vi "Translator.GatherControls.Prepare.vi"(8 "error in":errorcluster, 9 "root":string, 10 "Controls in":refnum<vi>[](array[refnum])) -> (0 "error out":errorcluster, 2 "Controls out":T1[](array[typedef]))   [LabVIEW 2016]
uses:
  Translator.ControlData.ctl
  Translator.ControlTypes.ctl
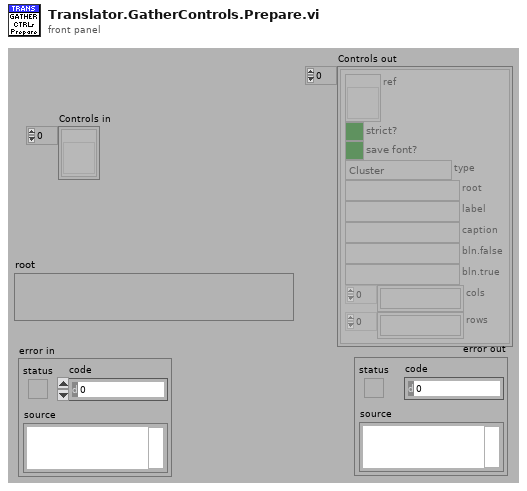
[diagram p1: front panel]
types:
  T1 = typedef "Translator.ControlData.ctl" = cluster{"ref":refnum<vi>, "strict?":bool, "save font?":bool, "type":T2, "root":string, "label":string, "caption":string, "bln.false":string, "bln.true":string, "cols":string[], "rows":string[]}
  T2 = typedef "Translator.ControlTypes.ctl" = enum16{"Cluster", "Array", "Boolean", "Ring", "String", "Tab", "Listbox", "Multicolumn listbox", "Table", "Tree", "Other"}
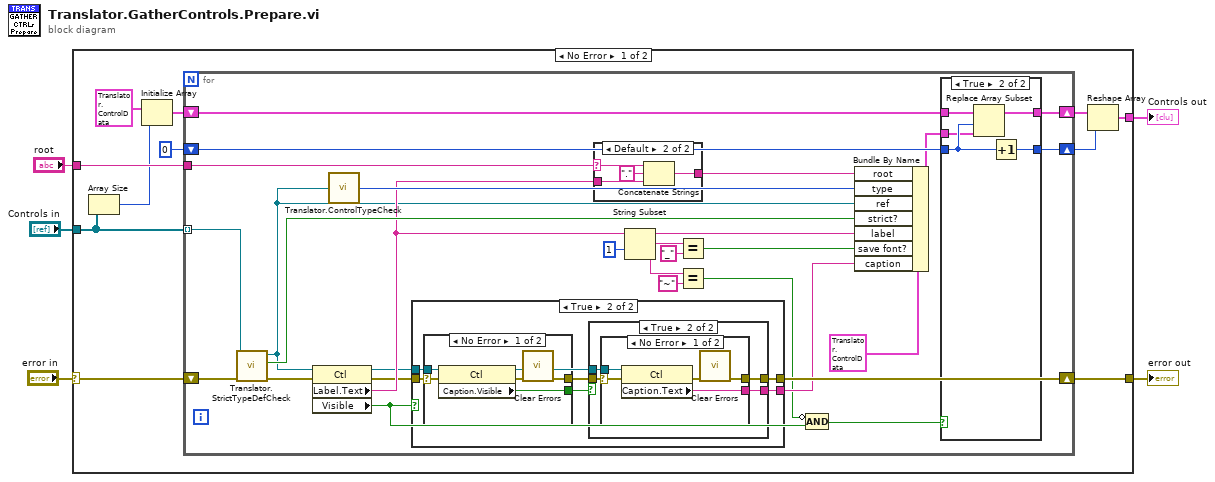
[diagram p0: block diagram]
diagram:
  n1 = case shown="No Error" "error in" {
    selector: "error in" -> [w15 w80]
    tunnel: "Controls in" -> [w13 _]
    tunnel: [w16 w80] -> w4
    tunnel: [w6 _] -> w3
    tunnel: "root" -> [w14 _]
    frame No Error {
      n2 = Array Size(array=w13) -> (size(s)=w11:i32)
      n3 = Initialize Array(T1 {"ref"=refnum, "strict?"=FALSE, "save font?"=FALSE, "type"=enum."Cluster", "root"="", "label"="", "caption"="", "bln.false"="", "bln.true"="", "cols"=[], "rows"=[]} ("ControlData"), w11) -> (w10:T1[])
      n4 = for {
        shift-right: [w41] -> w16
        shift-left: w15 -> [w40]
        tunnel: w13 -> [w37] mode=indexing
        tunnel: w14 -> [w35]
        shift-right: [w31] -> w8
        shift-left: w10 -> [w33]
        shift-right: [w30] -> w7
        shift-left: 0 -> [w32]
        n5 = call "Translator.StrictTypeDefCheck.vi"("error in (no error)"=w40, "Ctl Refnum in"=w37) -> ("error out"=w38:errorcluster, "Strict Type def?"=w39:bool, "Ctl Refnum out"=w21:refnum<vi>)  [unwired: 7 in]
        n6 = property class="Ctl"(reference=w21, error in=w38) -> (reference out=w23:refnum<vi>, error out=w24:errorcluster, "Label.Text"=w26:string, "Visible"=w22:bool)
        n7 = call "Translator.ControlTypeCheck.vi"("control ref"=w21) -> ("control type"=w42:T2)
        n8 = case shown="True" w22 {
          tunnel: [w44 w50] -> w41
          tunnel: [_ w49] -> w34
          tunnel: w24 -> [w44 w48]
          tunnel: w23 -> [_ w47]
          frame False {
          }
          frame True {
            n9 = case shown="No Error" w48 {
              selector: w48 -> [w66 w67]
              tunnel: [w63 w67] -> w46
              tunnel: w47 -> [w64 _]
              tunnel: [w62 _] -> w45
              frame No Error {
                n10 = property class="Ctl"(reference=w64, error in=w66) -> (error out=w65:errorcluster, "Caption.Visible"=w62:bool)  [unwired: 1 out]
                n11 = call <vilib>:"Clear Errors.vi"("error in (no error)"=w65) -> ("error out"=w63:errorcluster)  [unwired: 5 in, 1 out]
              }
              frame Error {
              }
            }
            n12 = case shown="True" w45 {
              tunnel: [w51 w55] -> w50
              tunnel: [_ w54] -> w49
              tunnel: w47 -> [_ w53]
              tunnel: w46 -> [w51 w52]
              frame False {
              }
              frame True {
                n13 = case shown="No Error" w52 {
                  selector: w52 -> [w60 w61]
                  tunnel: [w56 _] -> w54
                  tunnel: [w57 w61] -> w55
                  tunnel: w53 -> [w58 _]
                  frame No Error {
                    n14 = property class="Ctl"(reference=w58, error in=w60) -> (error out=w59:errorcluster, "Caption.Text"=w56:string)  [unwired: 1 out]
                    n15 = call <vilib>:"Clear Errors.vi"("error in (no error)"=w59) -> ("error out"=w57:errorcluster)  [unwired: 5 in, 1 out]
                  }
                  frame Error {
                  }
                }
              }
            }
          }
        }
        n16 = case shown="Default" w35 {
          selector: w35 -> [_ w76]
          tunnel: [w75 w79] -> w36
          tunnel: w26 -> [w75 w78]
          frame "" {
          }
          frame Default {
            n17 = Concatenate Strings(w76, "." ("string"), w78) -> (w79:string)
          }
        }
        n18 = String Subset(string=w26, length (rest)=1 ("length (rest)")) -> (substring=w18:string)  [unwired: 1 in]
        n19 = Equal?(x=w18, y="_") -> (x = y?=w25:bool)
        n20 = Equal?(x=w18, y="~") -> (x = y?=w17:bool)
        n21 = Compound Arithmetic op=AND(invert w17, w22) -> (w20:bool)
        n22 = Bundle By Name(cluster=T1 {"ref"=refnum, "strict?"=FALSE, "save font?"=FALSE, "type"=enum."Cluster", "root"="", "label"="", "caption"="", "bln.false"="", "bln.true"="", "cols"=[], "rows"=[]} ("ControlData"), "root"=w36, "type"=w42, "ref"=w21, "strict?"=w39, "label"=w26, "save font?"=w25, "caption"=w34) -> (w29:T1)
        n23 = case shown="True" w20 {
          tunnel: w33 -> [w68 w74]
          tunnel: w32 -> [w69 w72]
          tunnel: [w68 w73] -> w31
          tunnel: [w69 w71] -> w30
          tunnel: w29 -> [_ w70]
          frame False {
          }
          frame True {
            n24 = Replace Array Subset(array=w74, new element=w70, index=w72) -> (w73:T1[])
            n25 = Increment(x=w72) -> (x+1=w71:i32)
          }
        }
      }
      n26 = Reshape Array(w8, w7) -> (w6:T1[])
    }
    frame Error {
    }
  }
  "Controls out" <- w3
  "error out" <- w4
